vi "RSZVB Print to File.vi"(4 "Diagram Area (0: All Diagram Areas)":i32(ring) items=["All Diagram Areas", "Active Diagram Area", "Single Diagram Area"], 5 "Marker List (T: On)":bool=TRUE, 6 "Date and Time (T: On)":bool=TRUE, 7 "Logo (T: On)":bool=TRUE, 8 "error in (no error)":errorcluster {"code" format="%.0x"}, 9 "File Format (1: BMP)":i32(ring)=1 items=["EMF, EWMF", "BMP", "JPG", "PNG"], 10 "File Name (print-out.bmp)":string="print-out.bmp", 11 "VISA session":refnum<visa-resource-name>) -> (0 "error out":errorcluster {"code" format="%.0x"}, 3 "dup VISA session":refnum<visa-resource-name>)   [LabVIEW 2011]
doc: "This VI specify how the screen contents are stored to a file.\n\nDefines a name for a file which can be used to store the printer output. The file is created when it is selected as a printer destination (HCOPy:DESTination 'MMEM'). \n\nRemote-control command(s):\nMMEMory:NAME '<file_name>'\nHCOPy:DESTination 'MMEM'\nHCOPy:ITEM:ALL\nHCOPy:ITEM:LOGO[:STATe] <Boolean>\nHCOPy:ITEM:MLISt[:STATe] <Boolean>\nHCOPy:ITEM:TIME[:STATe] <Boolean>\nHCOPy:PAGE:WINDow ALL | ACTive | SINGle\nHCOPy:DEVice:LANGuage EMF | EWMF | BMP | PNG | JPG\nHCOPy[:IMMediate]"
panel:
  # "On\nOff"
  # "On\nOff"
  # "On\nOff"
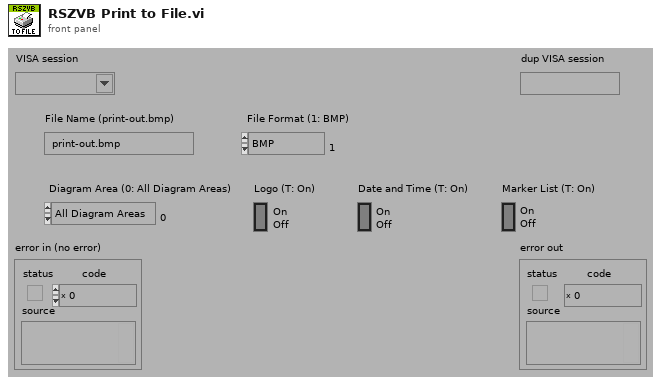
[diagram p1: front panel]
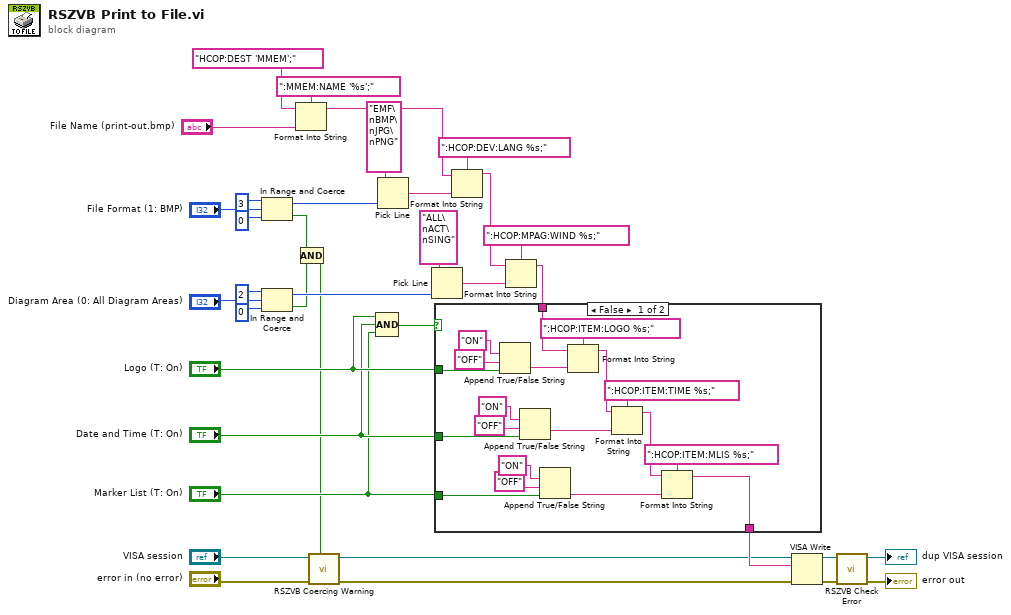
[diagram p0: block diagram]
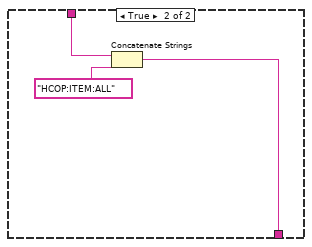
[diagram p2: hidden frame]
diagram:
  n1 = In Range and Coerce(upper limit=3, x="File Format (1: BMP)", lower limit=0) -> (coerced(x)=w13:i32, In Range?=w10:bool)
  n2 = In Range and Coerce(upper limit=2, x="Diagram Area (0: All Diagram Areas)", lower limit=0) -> (coerced(x)=w14:i32, In Range?=w9:bool)
  n3 = Format Into String(format string=":MMEM:NAME '%s';", initial string="HCOP:DEST 'MMEM';", "File Name (print-out.bmp)") -> (resulting string=w2:string)  [unwired: 1 in, 1 out]
  n4 = Compound Arithmetic op=AND(w10, w9) -> (w8:bool)
  n5 = call "RSZVB Coercing Warning.vi"("In Range?"=w8, "error in (no error)"="error in (no error)", "VISA session"="VISA session") -> ("error out"=w4:errorcluster, "dup VISA session"=w5:refnum<visa-resource-name>)  [unwired: 7 in]
  n6 = Compound Arithmetic op=AND("Logo (T: On)", "Date and Time (T: On)", "Marker List (T: On)") -> (w21:bool)
  n7 = Pick Line(multi-line string="EMF\nBMP\nJPG\nPNG", line index=w13) -> (output string=w30:string)  [unwired: 1 in]
  n8 = Pick Line(multi-line string="ALL\nACT\nSING", line index=w14) -> (output string=w25:string)  [unwired: 1 in]
  n9 = Format Into String(format string=":HCOP:DEV:LANG %s;", initial string=w2, w30) -> (resulting string=w3:string)  [unwired: 1 in, 1 out]
  n10 = Format Into String(format string=":HCOP:MPAG:WIND %s;", initial string=w3, w25) -> (resulting string=w20:string)  [unwired: 1 in, 1 out]
  n11 = case shown="False" w21 {
    tunnel: "Logo (T: On)" -> [w49 _]
    tunnel: "Date and Time (T: On)" -> [w48 _]
    tunnel: "Marker List (T: On)" -> [w47 _]
    tunnel: w20 -> [w38 w58]
    tunnel: [w37 w56] -> w19
    frame False {
      n12 = Append True/False String(1:w49, 2:"OFF", 3:"ON") -> (0:w43:string)  [unwired: 1 in]
      n13 = Append True/False String(1:w48, 2:"OFF", 3:"ON") -> (0:w42:string)  [unwired: 1 in]
      n14 = Append True/False String(1:w47, 2:"OFF", 3:"ON") -> (0:w41:string)  [unwired: 1 in]
      n15 = Format Into String(format string=":HCOP:ITEM:LOGO %s;", initial string=w38, w43) -> (resulting string=w40:string)  [unwired: 1 in, 1 out]
      n16 = Format Into String(format string=":HCOP:ITEM:TIME %s;", initial string=w40, w42) -> (resulting string=w39:string)  [unwired: 1 in, 1 out]
      n17 = Format Into String(format string=":HCOP:ITEM:MLIS %s;", initial string=w39, w41) -> (resulting string=w37:string)  [unwired: 1 in, 1 out]
    }
    frame True {
      n18 = Concatenate Strings(w58, "HCOP:ITEM:ALL") -> (w56:string)
    }
  }
  n19 = VISA Write(VISA resource name=w5, write buffer=w19, error in (no error)=w4) -> (VISA resource name out=w36:refnum<visa-resource-name>, error out=w35:errorcluster)  [unwired: 1 out]
  n20 = call "RSZVB Check Error.vi"("error in (no error)"=w35, "VISA session"=w36) -> ("error out"=→"error out":errorcluster, "dup VISA session"=→"dup VISA session":refnum<visa-resource-name>)  [unwired: 8 in]
